vi "Exporting_last_uploaded_settings_Core.vi"() -> ()   [LabVIEW 2011]
uses:
  common/typedefs/Waveforms_Cluster_Core.ctl
  common/typedefs/Unit_Names_Core.ctl
  common/typedefs/Data_Sources_Core.ctl
  common/typedefs/Types_of_Signals_Core.ctl
  common/typedefs/Types_of_Analyses_Core.ctl
  common/typedefs/Analysis_Parameters_Cluster_Core.ctl
  <vilib>/Analysis/3filter.llb/Filter Passband Type.ctl
  common/typedefs/Integration_Types_Core.ctl
  common/typedefs/Pan_Cluster_Core.ctl
  common/typedefs/Condition_Vector_Cluster_Core.ctl
  common/typedefs/cRIO_System_Settings_Cluster_Core.ctl
  common/typedefs/DSA_Channels_Configuration_Core.ctl
  <vilib>/addons/database/Connection.llb/DB Tools Open Connec (String).vi
  <vilib>/addons/database/Connection.llb/Conn Execute.vi
  <vilib>/addons/database/Recordset.llb/Rec Fetch Recordset Data (R).vi
  <vilib>/addons/database/Recordset.llb/Rec Destroy - Connection.vi
  <vilib>/addons/database/_DB Variant To Data/Database Variant To Data.xnode
  <vilib>/addons/database/NI_Database_API.lvlib
  <vilib>/Analysis/NI_AALBase.lvlib
panel:
  out "SettingsDescription (Always) 4":string
  out "Timestamp (Always) 4":dbl
  out "idtsettings (Always) 4":u32
  out "error out 10":errorcluster
  out "error out 9":errorcluster
  in  "cRIO system settings cluster 2":T1={"CONFIG Folder - Relative Path "=path "", "FIFO Depth (# of elements)"=0, "Avoid ALARM/ TRIP in transient regimes?"=FALSE, "Sample Rate [Hz]"=0.0, "Processing interval [s]"=0.0, "Total number of channels to read from FPGA  (auto-calculated)"=0, "# of data to read-DMA (auto-calculated)"=0, "SysLog Interval (s)"=0, "Running Log Folder - Relative Path "=path "Logs/Running_Log", "Reset Log File - Relative Path "=path "Logs/ResetLogs/cRIO_reset.txt", "Error Log File - Relative Path "=path "Logs/ErrLogs/Errlogs.txt", "Ring Buffer Size (# Log File Elements)"=86400, "CPU Usage Exceed Limit ()"=98.0, "CPU Usage Exceed Limit Delay (# of iterrations)"=60, "Free Memory Min Avail.  (%)"=15.0, "Base CoDiS Folder"=path "c:/CoDiS", "Archive Log Folder - Relative Path "=path "Logs/Archive_Log", "Avail. Drive Space Limit to do Archive (%)"=20.0, "Mediator IP address"="10.50.10.1", "Mediator Communication TCP/IP Port"=2055, "Used channels (from FPGA) per units -Auto calculated"=[], "# DMA FIFO Fulls File - Relative Path "=path "Logs/ResetLogs/cRIO_reset.txt", "Log Status Parameters in cRIO Ring Buffer"=FALSE, "Channels Input Configuration (has to be defined for all available AI)"=[], "Index to check OL and SC (from FPGA) per units and channels -Auto calculated)"=[], "System not OK? (Auto-calculated)"=FALSE, "System not OK Relay Number (-1 = none, 0,..., MAX)"=-1, "Use normal (T) or inverse (F) relay logic for given relay (size of array equals to number of relays)?"=[], "U32 Relay Output (Auto-calculated)"=0, "cRIO Source"=enum."Not Used", "Check DMA FIFO Full?"=FALSE, "Modbus Settings"={"Modbus Communication Port"=502, "Run as Modbus Server/Slave? (FALSE=Modbus Client/Master)"=FALSE, "Modbus Slave Remote IP Address (if Run as Modbus Server/Slave?=FALSE)"=""}, "Time Synchronization Settings"={"Enable Time Synchronization"=FALSE, "Time Server IP Address (if Enable Time Synchronization=TRUE)"=""}} {"Channels Input Configuration (has to be defined for all available AI)" items=["AC Coupled", "DC Coupled", "IEPE AC Coupled", "Not DSA Channel"]}
  in  "cRIO system settings cluster":T1={"CONFIG Folder - Relative Path "=path "", "FIFO Depth (# of elements)"=0, "Avoid ALARM/ TRIP in transient regimes?"=FALSE, "Sample Rate [Hz]"=0.0, "Processing interval [s]"=0.0, "Total number of channels to read from FPGA  (auto-calculated)"=0, "# of data to read-DMA (auto-calculated)"=0, "SysLog Interval (s)"=0, "Running Log Folder - Relative Path "=path "Logs/Running_Log", "Reset Log File - Relative Path "=path "Logs/ResetLogs/cRIO_reset.txt", "Error Log File - Relative Path "=path "Logs/ErrLogs/Errlogs.txt", "Ring Buffer Size (# Log File Elements)"=86400, "CPU Usage Exceed Limit ()"=98.0, "CPU Usage Exceed Limit Delay (# of iterrations)"=60, "Free Memory Min Avail.  (%)"=15.0, "Base CoDiS Folder"=path "c:/CoDiS", "Archive Log Folder - Relative Path "=path "Logs/Archive_Log", "Avail. Drive Space Limit to do Archive (%)"=20.0, "Mediator IP address"="10.50.10.1", "Mediator Communication TCP/IP Port"=2055, "Used channels (from FPGA) per units -Auto calculated"=[], "# DMA FIFO Fulls File - Relative Path "=path "Logs/ResetLogs/cRIO_reset.txt", "Log Status Parameters in cRIO Ring Buffer"=FALSE, "Channels Input Configuration (has to be defined for all available AI)"=[], "Index to check OL and SC (from FPGA) per units and channels -Auto calculated)"=[], "System not OK? (Auto-calculated)"=FALSE, "System not OK Relay Number (-1 = none, 0,..., MAX)"=-1, "Use normal (T) or inverse (F) relay logic for given relay (size of array equals to number of relays)?"=[], "U32 Relay Output (Auto-calculated)"=0, "cRIO Source"=enum."Not Used", "Check DMA FIFO Full?"=FALSE, "Modbus Settings"={"Modbus Communication Port"=502, "Run as Modbus Server/Slave? (FALSE=Modbus Client/Master)"=FALSE, "Modbus Slave Remote IP Address (if Run as Modbus Server/Slave?=FALSE)"=""}, "Time Synchronization Settings"={"Enable Time Synchronization"=FALSE, "Time Server IP Address (if Enable Time Synchronization=TRUE)"=""}} {"Channels Input Configuration (has to be defined for all available AI)" items=["AC Coupled", "DC Coupled", "IEPE AC Coupled", "Not DSA Channel"]}
  in  "Pan Cluster":T4={"Configuration File loaded successfully?"=FALSE, "Is this new configuration?"=FALSE, "Condition Vector Cluster"={"Unit Name"=enum."Unit 2", "Source Name"=[], "Use CoDiS server Timestamp (on FALSE uses Processing Unit Timestamp)?"=FALSE, "Timestamp (DBL)"=0.0, "Mode of Operation - Normal (Settings)"=[], "Mode of Operation - Normal"="", "Mode of Operation - Diagnostic (Settings)"=[], "Mode of Operation - Diagnostic Recognized Index"=0, "Condition Vector Label"=[], "Condition Vector Name"=[], "Is this Main Trigger Signal?"=[], "Perform PRE-ALARM, ALARM, etc. Analysis on CoDiS server (mediator main calc. loop)?"=[], "Trigger Indexes"=[], "Condition Vector Values Complex (CDB)"=[], "Condition Vector Values"=[], "Save to dBase"=[], "Check if Condition Vector Element is out of Range"=[], "Condition Vector Low Limit Value"=[], "Condition Vector High Limit Value"=[], "Condition Vector Element out of Range"=[], "Check for PRE-ALARM"=[], "PRE-ALARM Value"=[], "Number of Loops in PRE-ALARM"=[], "PRE-ALARM Delay in # of Loops"=[], "Is Value Increasing for PRE-ALARM?"=[], "In PRE-ALARM?"=[], "In Delayed PRE-ALARM?"=[], "In Delayed PRE-ALARM REM?"=[], "Save PRE-ALARM?"=FALSE, "Check for ALARM"=[], "ALARM Value"=[], "Number of Loops in ALARM"=[], "ALARM Delay in # of Loops"=[], "Is Value Increasing for ALARM?"=[], "In ALARM?"=[], "In Delayed ALARM?"=[], "In Delayed ALARM REM?"=[], "Save ALARM?"=FALSE, "ALARM Relay Number (-1 = none, 0, ..., MAX)"=[], "Check for PRE-TRIP"=[], "PRE-TRIP Value"=[], "Number of Loops in PRE-TRIP"=[], "PRE-TRIP Delay in # of Loops"=[], "Is Value Increasing for PRE-TRIP?"=[], "In PRE-TRIP?"=[], "In Delayed PRE-TRIP?"=[], "In Delayed PRE-TRIP REM?"=[], "Save PRE-TRIP?"=FALSE, "Check for TRIP"=[], "TRIP Value"=[], "Number of Loops in TRIP"=[], "TRIP Delay in # of Loops"=[], "Is Value Increasing for TRIP?"=[], "In TRIP?"=[], "In Delayed TRIP?"=[], "In Delayed TRIP REM?"=[], "Save TRIP?"=FALSE, "TRIP Relay Number(-1 = none, 0,..., MAX)"=[], "Check for Diagnostic ALARM"=[], "ZERO Machine Signature Value"=[], "Number of Loops in Diagnostic ALARM"=[], "Diagnostic ALARM Delay in # of Loops"=[], "Is Value Increasing for Diagnostic ALARM?"=[], "In Diagnostic ALARM?"=[], "In Delayed Diagnostic ALARM?"=[], "In Delayed Diagnostic ALARM REM?"=[], "Save Diagnostic ALARM?"=FALSE, "Current Diagnostic Alarm Level"=[], "Delta for Diagnostic ALARM"=[], "Trigger RS for this channel?"=[], "Delta for RS Trigger"=[], "Modbus Parameters"={"Type"=[], "Modbus register"=[], "Which element type"=[], "Starting address"=[], "How many registers"=[], "Multiplication factor"=[]}, "Filter State"=[], "Apply Formula?"=[], "Formula Settings (If Apply Formula?=TRUE)"=[]}, "Orbit(s) - XY"=[], "Air Gap Data"=[], "Magnetic Field Data"=[], "Absolute Minimum Air Gap per Plane"=[]} {"Absolute Minimum Air Gap per Plane"."Absolute AG Minimum Pole Number" format="%.3f"; "Absolute Minimum Air Gap per Plane"."Absolute AG Minimum Value" format="%.3f"; "Magnetic Field Data"."Maximum by Pole Number" format="%.3f"; "Air Gap Data"."Minimum by Pole Number" format="%.3f"; "Orbit(s) - XY"."Orbit XY Graphs (Synthesized from Selected Harmonics and DC)"."?" format="%.3f"; "Orbit(s) - XY"."Orbit XY Graphs (Synthesized from Selected Harmonics and DC)"."?" format="%.3f"; "Orbit(s) - XY"."Orbit XY Graphs (Glided and Averaged on One Revolution)"."?" format="%.3f"; "Orbit(s) - XY"."Orbit XY Graphs (Glided and Averaged on One Revolution)"."?" format="%.3f"; "Orbit(s) - XY"."Orbit XY Graphs (Unaveraged)"."?" format="%.3f"; "Orbit(s) - XY"."Orbit XY Graphs (Unaveraged)"."?" format="%.3f"}
  out "error out 6":errorcluster
  out "error out 5":errorcluster
  out "idtsettings (Always) 3":u32
  out "Timestamp (Always) 3":dbl
  out "SettingsDescription (Always) 3":string
  out "error out 4":errorcluster
  out "error out 3":errorcluster
  out "idtsettings (Always) 2":u32
  out "Timestamp (Always) 2":dbl
  out "SettingsDescription (Always) 2":string
  out "error out 2":errorcluster
  out "error out":errorcluster
  in  "Empty Waveform Cluster":T7={"Configuration File loaded successfully? "=FALSE, "Is this new configuration?"=FALSE, "Unit Name"=enum."Unit 1", "Waveform Source"=[], "Use CoDiS server Timestamp (on FALSE uses Processing Unit Timestamp)?"=FALSE, "Sampling Rate [Hz]"=[], "Timestamp (DBL)"=0.0, "Mode of Operation - Normal"="", "Mode of Operation - Diagnostic"="", "Waveform Physical Channel"=[], "Waveform Label"=[], "Waveform Name"=[], "Signal Type"=[], "Is this Main Trigger Signal?"=[], "Slope"=[], "Intercept"=[], "Waveform Values"=[], "Analyse?"=[], "Save to database?"=[], "Analyses to Perform"=[], "Perform this analysis on a CoDiS server?"=[], "General Parameters"={"Number of Poles"=0, "Grid Frequency"=0.0}, "Analysis Parameters"=[], "Save now to dBase?"=FALSE, "Waveform Length for Saving [s]"=0, "Pretrigger Length when Saving Waveform [s]"=0, "Next Timestamp to autosave at (DBL)"=0.0, "Description of Waveforms Events"="", "Event Type"="", "Save next RS event entirely? (on FALSE uses How many basic (acquisition) blocks of data (loops) to save?"=FALSE, "Regime Name for which to save next RS event entirely"="", "Integration type"=[], "Channel not OK?"=[], "Channel Not OK?  Relay Number (-1 = none, 0, ..., MAX)"=[], "Array of FPGA Filter Parameters"=[], "Pre-Alarm Delay in Number of Loops "=0, "Pre-Trip Delay in Number of Loops "=0} {"Analysis Parameters"."SP2Pmax"."Filter Parameters"."low cutoff freq: fl" format="%0.4f"; "Analysis Parameters"."SP2Pmax"."Filter Parameters"."high cutoff freq: fh" format="%0.2f"; "Analysis Parameters"."LoadAngleDelta"."Multiplication Factor" format="%.1f"; "Analysis Parameters"."LoadAngleDelta"."What harmonic? (for example 24th (48 pole machine))" format="%.1f"; "Analysis Parameters"."Peak2Peak"."Filter Parameters"."low cutoff freq: fl" format="%0.4f"; "Analysis Parameters"."Peak2Peak"."Filter Parameters"."high cutoff freq: fh" format="%0.2f"; "Analysis Parameters"."RMS"."Filter Parameters"."order" format="%0.4f"; "Analysis Parameters"."RMS"."Filter Parameters"."low cutoff freq: fl" format="%0.2f"; "Analysis Parameters"."RMS"."Filter Parameters"."high cutoff freq: fh" format="%0.2f"; "Analysis Parameters"."EqPeak"."Filter Parameters"."low cutoff freq: fl" format="%0.4f"; "Analysis Parameters"."EqPeak"."Filter Parameters"."high cutoff freq: fh" format="%0.2f"; "Analysis Parameters"."Peak"."Filter Parameters"."low cutoff freq: fl" format="%0.4f"; "Analysis Parameters"."Peak"."Filter Parameters"."high cutoff freq: fh" format="%0.2f"; "Analysis Parameters"."snPh"."What harmonic?" format="%.1f"; "Analysis Parameters"."snA"."Multiplication Factor" format="%.1f"; "Analysis Parameters"."snA"."What harmonic?" format="%.1f"; "Analysis Parameters"."Smax"."Filter Parameters"."low cutoff freq: fl" format="%0.4f"; "Analysis Parameters"."Smax"."Filter Parameters"."high cutoff freq: fh" format="%0.2f"; "Analysis Parameters"."RPM"."Signal Threshold" format="%.1f"}
  out "idtsettings (Always)":u32
  out "Timestamp (Always)":dbl
  out "SettingsDescription (Always)":string
  out "Waveform Cluster (Depending on Selection)":T7={"Configuration File loaded successfully? "=FALSE, "Is this new configuration?"=FALSE, "Unit Name"=enum."Unit 1", "Waveform Source"=[], "Use CoDiS server Timestamp (on FALSE uses Processing Unit Timestamp)?"=FALSE, "Sampling Rate [Hz]"=[], "Timestamp (DBL)"=0.0, "Mode of Operation - Normal"="", "Mode of Operation - Diagnostic"="", "Waveform Physical Channel"=[], "Waveform Label"=[], "Waveform Name"=[], "Signal Type"=[], "Is this Main Trigger Signal?"=[], "Slope"=[], "Intercept"=[], "Waveform Values"=[], "Analyse?"=[], "Save to database?"=[], "Analyses to Perform"=[], "Perform this analysis on a CoDiS server?"=[], "General Parameters"={"Number of Poles"=0, "Grid Frequency"=0.0}, "Analysis Parameters"=[], "Save now to dBase?"=FALSE, "Waveform Length for Saving [s]"=0, "Pretrigger Length when Saving Waveform [s]"=0, "Next Timestamp to autosave at (DBL)"=0.0, "Description of Waveforms Events"="", "Event Type"="", "Save next RS event entirely? (on FALSE uses How many basic (acquisition) blocks of data (loops) to save?"=FALSE, "Regime Name for which to save next RS event entirely"="", "Integration type"=[], "Channel not OK?"=[], "Channel Not OK?  Relay Number (-1 = none, 0, ..., MAX)"=[], "Array of FPGA Filter Parameters"=[], "Pre-Alarm Delay in Number of Loops "=0, "Pre-Trip Delay in Number of Loops "=0} {"Analysis Parameters"."SP2Pmax"."Filter Parameters"."low cutoff freq: fl" format="%0.4f"; "Analysis Parameters"."SP2Pmax"."Filter Parameters"."high cutoff freq: fh" format="%0.2f"; "Analysis Parameters"."LoadAngleDelta"."Multiplication Factor" format="%.1f"; "Analysis Parameters"."LoadAngleDelta"."What harmonic? (for example 24th (48 pole machine))" format="%.1f"; "Analysis Parameters"."Peak2Peak"."Filter Parameters"."low cutoff freq: fl" format="%0.4f"; "Analysis Parameters"."Peak2Peak"."Filter Parameters"."high cutoff freq: fh" format="%0.2f"; "Analysis Parameters"."RMS"."Filter Parameters"."order" format="%0.4f"; "Analysis Parameters"."RMS"."Filter Parameters"."low cutoff freq: fl" format="%0.2f"; "Analysis Parameters"."RMS"."Filter Parameters"."high cutoff freq: fh" format="%0.2f"; "Analysis Parameters"."EqPeak"."Filter Parameters"."low cutoff freq: fl" format="%0.4f"; "Analysis Parameters"."EqPeak"."Filter Parameters"."high cutoff freq: fh" format="%0.2f"; "Analysis Parameters"."Peak"."Filter Parameters"."low cutoff freq: fl" format="%0.4f"; "Analysis Parameters"."Peak"."Filter Parameters"."high cutoff freq: fh" format="%0.2f"; "Analysis Parameters"."snPh"."What harmonic?" format="%.1f"; "Analysis Parameters"."snA"."Multiplication Factor" format="%.1f"; "Analysis Parameters"."snA"."What harmonic?" format="%.1f"; "Analysis Parameters"."Smax"."Filter Parameters"."low cutoff freq: fl" format="%0.4f"; "Analysis Parameters"."Smax"."Filter Parameters"."high cutoff freq: fh" format="%0.2f"; "Analysis Parameters"."RPM"."Signal Threshold" format="%.1f"}
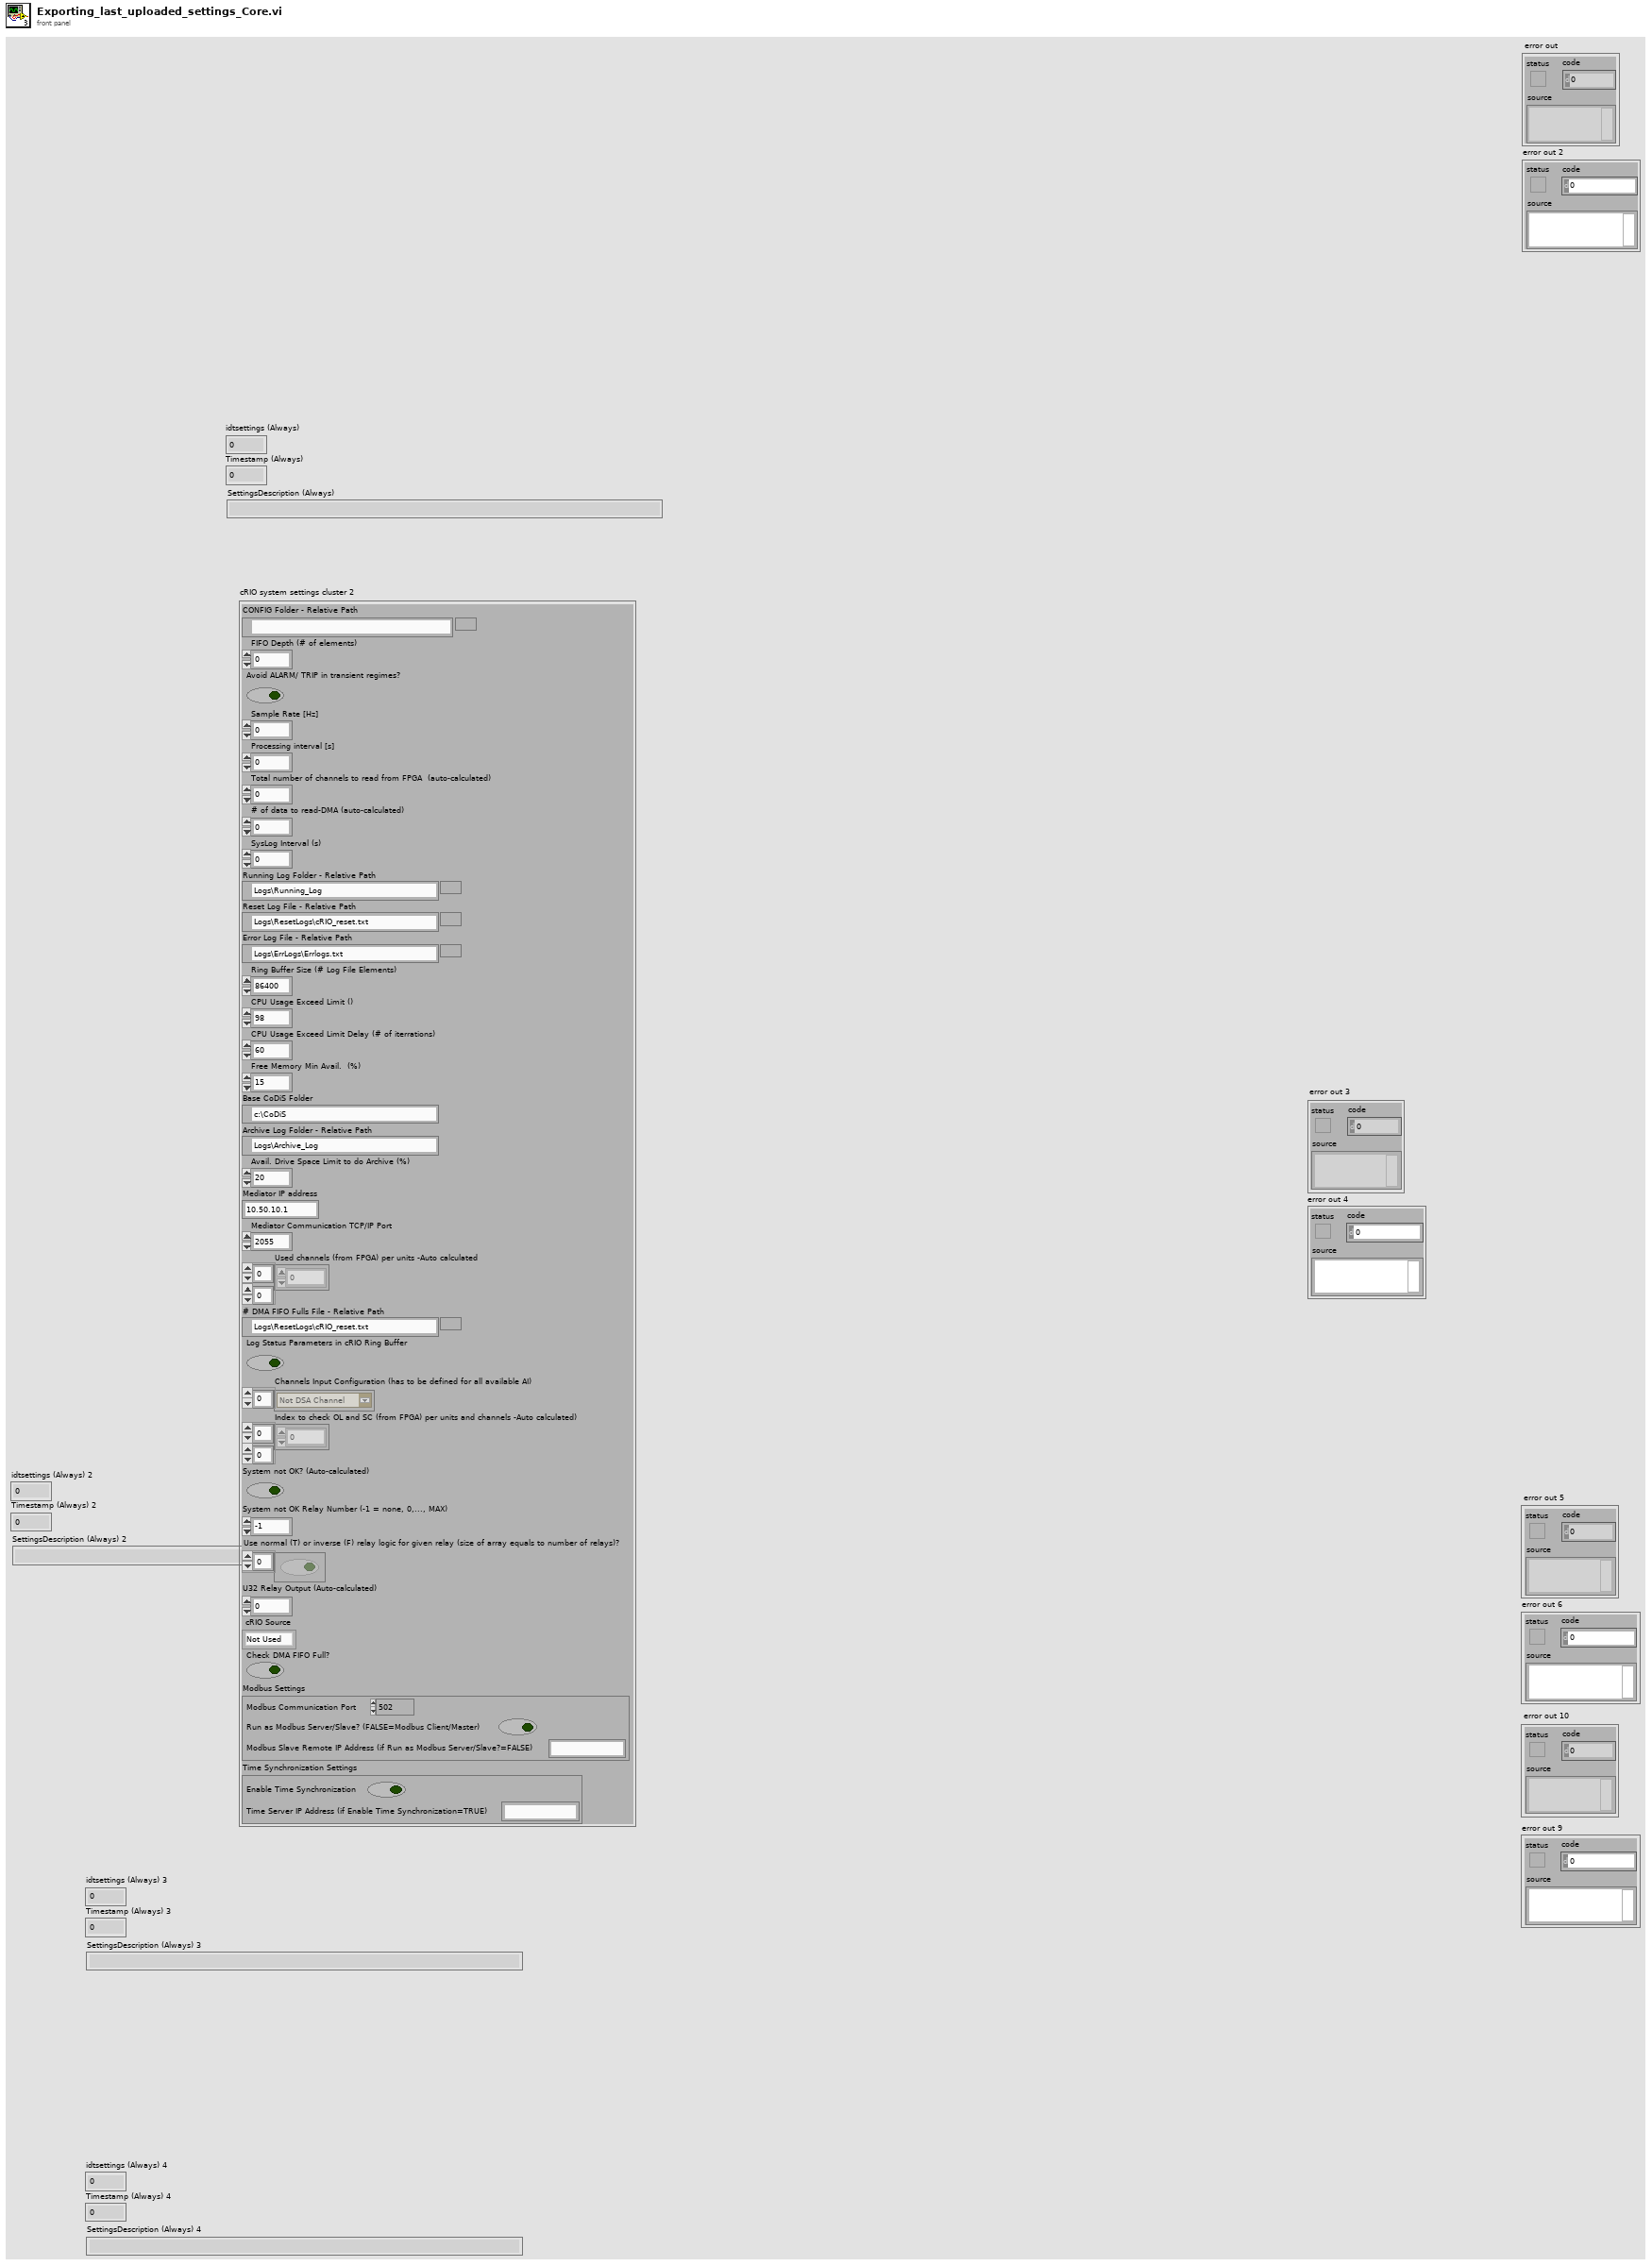
[diagram p1: front panel]
types:
  T1 = typedef "cRIO_System_Settings_Cluster_Core.ctl" = cluster{"CONFIG Folder - Relative Path ":path, "FIFO Depth (# of elements)":u32, "Avoid ALARM/ TRIP in transient regimes?":bool, "Sample Rate [Hz]":sgl, "Processing interval [s]":sgl, "Total number of channels to read from FPGA  (auto-calculated)":u32, "# of data to read-DMA (auto-calculated)":u32, "SysLog Interval (s)":u32, "Running Log Folder - Relative Path ":path, "Reset Log File - Relative Path ":path, "Error Log File - Relative Path ":path, "Ring Buffer Size (# Log File Elements)":u32, "CPU Usage Exceed Limit ()":sgl, "CPU Usage Exceed Limit Delay (# of iterrations)":u32, "Free Memory Min Avail.  (%)":sgl, "Base CoDiS Folder":path, "Archive Log Folder - Relative Path ":path, "Avail. Drive Space Limit to do Archive (%)":sgl, "Mediator IP address":string, "Mediator Communication TCP/IP Port":u16, "Used channels (from FPGA) per units -Auto calculated":i32[][], "# DMA FIFO Fulls File - Relative Path ":path, "Log Status Parameters in cRIO Ring Buffer":bool, "Channels Input Configuration (has to be defined for all available AI)":T2[], "Index to check OL and SC (from FPGA) per units and channels -Auto calculated)":i32[][], "System not OK? (Auto-calculated)":bool, "System not OK Relay Number (-1 = none, 0,..., MAX)":i16, "Use normal (T) or inverse (F) relay logic for given relay (size of array equals to number of relays)?":bool[], "U32 Relay Output (Auto-calculated)":u32, "cRIO Source":T3, "Check DMA FIFO Full?":bool, "Modbus Settings":cluster{"Modbus Communication Port":u16, "Run as Modbus Server/Slave? (FALSE=Modbus Client/Master)":bool, "Modbus Slave Remote IP Address (if Run as Modbus Server/Slave?=FALSE)":string}, "Time Synchronization Settings":cluster{"Enable Time Synchronization":bool, "Time Server IP Address (if Enable Time Synchronization=TRUE)":string}}
  T2 = typedef "DSA_Channels_Configuration_Core.ctl" = u16
  T3 = typedef "Data_Sources_Core.ctl" = enum16{"Not Used", "Source 0", "Source 1", "Source 2", "Source 3", "Source 4", "Source 5", "Source 6", "Source 7", "Source 8", "Source 9", "Source 10", "Source 11", "Source 12", "Source 13", "Source 14", "Source 15", "Source 16", "Source 17", "Source 18", "Source 19", "Source 20"}
  T4 = typedef "Pan_Cluster_Core.ctl" = cluster{"Configuration File loaded successfully?":bool, "Is this new configuration?":bool, "Condition Vector Cluster":T5, "Orbit(s) - XY":cluster{"Bearing Plane Label (for example RV000&RV001 or RV001&RV000; 1st label is X, second is Y)":string, "Bearing Plane Name (for client purposes)":string, "Orbit XY Graphs (Unaveraged)":cluster{sgl[], sgl[]}[], "Glided and Averaged on One Revolution Parameters Cluster":cluster{"Calculate from time-averaged signal on one revolution?":bool, "Analyze data from 1st trigger to last (if possible)? (FALSE=analyze everything)":bool, "Gliding Parameters":cluster{"Glide signal?":bool, "Number of points for gliding":u16}}, "Orbit XY Graphs (Glided and Averaged on One Revolution)":cluster{sgl[], sgl[]}[], "Orbit XY Graphs (Synthesized from Selected Harmonics and DC)":cluster{sgl[], sgl[]}[], "Rotate Coordinate System?":bool, "Angle for rot. (if Rotate Coordinate System?=TRUE; angle is >0 for CCW, <0 for CW - view from generator (above for vert. mach.) side)":sgl}[], "Air Gap Data":cluster{"Air Gap Label":string, "Minimum by Pole Number":sgl[]}[], "Magnetic Field Data":cluster{"Magnetic Field Label":string, "Maximum by Pole Number":sgl[]}[], "Absolute Minimum Air Gap per Plane":cluster{"Air Gap Plane Name":string, "Air Gap Sensor Labels per Plane":string[], "Air Gap Sensor Name per Plane":string[], "Absolute AG Minimum Value":sgl, "Absolute AG Minimum Pole Number":sgl, "Absolute AG Minimum Sensor Label":string, "Absolute AG Minimum Sensor Name":string}[]}
  T5 = typedef "Condition_Vector_Cluster_Core.ctl" = cluster{"Unit Name":T6, "Source Name":T3[], "Use CoDiS server Timestamp (on FALSE uses Processing Unit Timestamp)?":bool, "Timestamp (DBL)":dbl, "Mode of Operation - Normal (Settings)":cluster{"Regime Name":string, "Regime Logical Definition Statement":string}[], "Mode of Operation - Normal":string, "Mode of Operation - Diagnostic (Settings)":cluster{"Regime Name":string, "Regime Logical Definition Statement":string}[], "Mode of Operation - Diagnostic Recognized Index":i16, "Condition Vector Label":string[], "Condition Vector Name":string[], "Is this Main Trigger Signal?":bool[], "Perform PRE-ALARM, ALARM, etc. Analysis on CoDiS server (mediator main calc. loop)?":bool[], "Trigger Indexes":u32[], "Condition Vector Values Complex (CDB)":cdb[], "Condition Vector Values":sgl[], "Save to dBase":bool[], "Check if Condition Vector Element is out of Range":bool[], "Condition Vector Low Limit Value":sgl[], "Condition Vector High Limit Value":sgl[], "Condition Vector Element out of Range":bool[], "Check for PRE-ALARM":bool[][], "PRE-ALARM Value":sgl[][], "Number of Loops in PRE-ALARM":u32[], "PRE-ALARM Delay in # of Loops":u16[][], "Is Value Increasing for PRE-ALARM?":bool[], "In PRE-ALARM?":bool[], "In Delayed PRE-ALARM?":bool[], "In Delayed PRE-ALARM REM?":bool[], "Save PRE-ALARM?":bool, "Check for ALARM":bool[][], "ALARM Value":sgl[][], "Number of Loops in ALARM":u32[], "ALARM Delay in # of Loops":u16[][], "Is Value Increasing for ALARM?":bool[], "In ALARM?":bool[], "In Delayed ALARM?":bool[], "In Delayed ALARM REM?":bool[], "Save ALARM?":bool, "ALARM Relay Number (-1 = none, 0, ..., MAX)":i16[], "Check for PRE-TRIP":bool[][], "PRE-TRIP Value":sgl[][], "Number of Loops in PRE-TRIP":u32[], "PRE-TRIP Delay in # of Loops":u16[][], "Is Value Increasing for PRE-TRIP?":bool[], "In PRE-TRIP?":bool[], "In Delayed PRE-TRIP?":bool[], "In Delayed PRE-TRIP REM?":bool[], "Save PRE-TRIP?":bool, "Check for TRIP":bool[][], "TRIP Value":sgl[][], "Number of Loops in TRIP":u32[], "TRIP Delay in # of Loops":u16[][], "Is Value Increasing for TRIP?":bool[], "In TRIP?":bool[], "In Delayed TRIP?":bool[], "In Delayed TRIP REM?":bool[], "Save TRIP?":bool, "TRIP Relay Number(-1 = none, 0,..., MAX)":i16[], "Check for Diagnostic ALARM":bool[][], "ZERO Machine Signature Value":dbl[][], "Number of Loops in Diagnostic ALARM":u32[], "Diagnostic ALARM Delay in # of Loops":u16[][], "Is Value Increasing for Diagnostic ALARM?":bool[], "In Diagnostic ALARM?":bool[], "In Delayed Diagnostic ALARM?":bool[], "In Delayed Diagnostic ALARM REM?":bool[], "Save Diagnostic ALARM?":bool, "Current Diagnostic Alarm Level":sgl[][], "Delta for Diagnostic ALARM":sgl[][], "Trigger RS for this channel?":bool[][], "Delta for RS Trigger":sgl[][], "Modbus Parameters":cluster{"Type":enum16{"Read", "Write", "None"}[][], "Modbus register":enum16{"Coils", "Discrete Inputs", "Input Registers", "Holding Registers"}[][], "Which element type":enum16{"Value", "Alarm", "Trip"}[][], "Starting address":u16[][], "How many registers":enum16{"Single register", "HI-LO", "LO-HI"}[][], "Multiplication factor":dbl[][]}, "Filter State":cluster{"Filter State (channels by rows: 0. ch0, 1. ch1, etc))":dbl[][]}[], "Apply Formula?":bool[][], "Formula Settings (If Apply Formula?=TRUE)":cluster{"Variables by Condition vector label (Example (array):  0. PROC000.DC; 1.PROC001.DC000)":string[], "Formula (example: (PROC000.DC+PROC001.DC000)/2  )":string}[][]}
  T6 = typedef "Unit_Names_Core.ctl" = enum16{"Not used", "Unit 1", "Unit 2", "Unit 3", "Unit 4", "Unit 5", "Unit 6", "Unit 7", "Unit 8", "Unit 9"}
  T7 = typedef "Waveforms_Cluster_Core.ctl" = cluster{"Configuration File loaded successfully? ":bool, "Is this new configuration?":bool, "Unit Name":T6, "Waveform Source":T3[], "Use CoDiS server Timestamp (on FALSE uses Processing Unit Timestamp)?":bool, "Sampling Rate [Hz]":u32[], "Timestamp (DBL)":dbl, "Mode of Operation - Normal":string, "Mode of Operation - Diagnostic":string, "Waveform Physical Channel":u16[], "Waveform Label":string[], "Waveform Name":string[], "Signal Type":cluster{"Signal Type":T8, "# of signal of particular type":u8}[], "Is this Main Trigger Signal?":bool[], "Slope":dbl[], "Intercept":dbl[], "Waveform Values":sgl[][], "Analyse?":bool[], "Save to database?":bool[], "Analyses to Perform":T9[][], "Perform this analysis on a CoDiS server?":bool[][], "General Parameters":cluster{"Number of Poles":u8, "Grid Frequency":sgl}, "Analysis Parameters":T10[][], "Save now to dBase?":bool, "Waveform Length for Saving [s]":u16, "Pretrigger Length when Saving Waveform [s]":u16, "Next Timestamp to autosave at (DBL)":dbl, "Description of Waveforms Events":string, "Event Type":string, "Save next RS event entirely? (on FALSE uses How many basic (acquisition) blocks of data (loops) to save?":bool, "Regime Name for which to save next RS event entirely":string, "Integration type":T12[], "Channel not OK?":bool[], "Channel Not OK?  Relay Number (-1 = none, 0, ..., MAX)":i16[], "Array of FPGA Filter Parameters":cluster{"Filter signal?":bool, "filter type":T11, "high cutoff freq: fh":dbl, "low cutoff freq: fl":dbl, "order":i32}[][], "Pre-Alarm Delay in Number of Loops ":u16, "Pre-Trip Delay in Number of Loops ":u16}
  T8 = typedef "Types_of_Signals_Core.ctl" = enum16{"Not Used", "Trigger (TRG???)", "Relative Vibrations (RV???)", "Absolute Vibrations (AV???)", "Air Gap (AG???)", "Magnetic Field (MX???)", "Voltage (VOL???)", "Current (CURR???)", "Process (PROC???)", "Cavitation (CAV???)", "Non Standard (NONST???)", "Axial Displacement (AXD???)", "Absolute Vibrations Stator Core (AVSC???)"}
  T9 = typedef "Types_of_Analyses_Core.ctl" = enum16{"Exit Analysis Loop", "Do Nothing", "RPM", "Smax", "SP2Pmax", "snA", "snPh", "Rest", "Peak", "EqPeak", "Peak2Peak", "RMS", "DC", "DC from Extrema", "Min Value", "Max Value", "Min Value by Pole", "Max Value by Pole", "Max Diff by Pole", "Max Diff Pole Number", "Min from Extrema", "Max from Extrema", "Active Power from DFT", "Active Power by Integration", "Reactive Power from DFT", "Reactive Power by Integration", "Apparent Power", "Ampl@Freq", "Phase Difference", "Load Angle Delta", "THD", "Signal Frequency", "Eta", "Non standard (CoDiS server - manual) 0", "Non standard (CoDiS server - manual) 1", "Non standard (CoDiS server - manual) 2", "Non standard (CoDiS server - manual) 3", "Non standard (CoDiS server - manual) 4", "Non standard (CoDiS server - manual) 5", "Non standard (CoDiS server - manual) 6", "Non standard (CoDiS server - manual) 7", "Non standard (CoDiS server - manual) 8", "Non standard (CoDiS server - manual) 9", "Non standard (CoDiS server - manual) 10", "Non standard (CoDiS server - manual) 11", "Non standard (CoDiS server - manual) 12", "Non standard (CoDiS server - manual) 13", "Non standard (CoDiS server - manual) 14", "Non standard (CoDiS server - manual) 15", "Non standard (CoDiS server - manual) 16", "Non standard (CoDiS server - manual) 17", "Non standard (CoDiS server - manual) 18", "Non standard (CoDiS server - manual) 19", "CosFi", "Total THD", "Crest Factor"}
  T10 = typedef "Analysis_Parameters_Cluster_Core.ctl" = cluster{"DC":cluster{"Analyze data from 1st trigger to last (if possible)? (FALSE=analyze everything)":bool}, "DCExtrema":cluster{"Calculate DC from all Pole Values":bool, "Poles to use in DC calculation (if Calculate DC from all Pole Values is FALSE)":u8[], "Condition Vector Label begin Part (MinPole or MaxPole)":string, "Addition to Condition Vector Label (example: 000)":string}, "RPM":cluster{"Signal Threshold":sgl, "Pulse Width (should be >= 2 depending on signal noise)":i32, "Trigger on rising edge? (FALSE=trigger on falling)":bool}, "Smax":cluster{"Combine with which Waveform Label? (for example: RV001)":string, "Calculate from time-averaged signal on one revolution?":bool, "Analyze data from 1st trigger to last (if possible)? (FALSE=analyze everything)":bool, "Filter Parameters":cluster{"Filter signal?":bool, "filter type":T11, "high cutoff freq: fh":dbl, "low cutoff freq: fl":dbl, "order":i32, "Process as ring-buffer signal?":bool}, "Gliding Parameters":cluster{"Glide signal?":bool, "Number of points for gliding":u16}, "Average all calculated values for Smax - if present (each revolution)? (FALSE=take absolute maximum)":bool, "Addition to Condition Vector Label (example: 000)":string}, "SP2Pmax":cluster{"Combine with which Waveform Label? (for example: RV001)":string, "Calculate from time-averaged signal on one revolution?":bool, "Analyze data from 1st trigger to last (if possible)? (FALSE=analyze everything)":bool, "Filter Parameters":cluster{"Filter signal?":bool, "filter type":T11, "high cutoff freq: fh":dbl, "low cutoff freq: fl":dbl, "order":i32, "Process as ring-buffer signal?":bool}, "Gliding Parameters":cluster{"Glide signal?":bool, "Number of points for gliding":u16}, "Average all calculated values for SP2Pmax - if present (each revolution)? (FALSE=take absolute maximum)":bool, "Addition to Condition Vector Label (example: 000)":string}, "snA":cluster{"What harmonic?":sgl, "Calculate Amplitude (TRUE) or RMS (FALSE)?":bool, "Multiplication Factor":sgl, "Calculate Amplitude for Air Gap type signals? (from MinPole Values)":bool}, "snPh":cluster{"What harmonic?":sgl}, "Peak":cluster{"Calculate from time-averaged signal (one-revolution)?":bool, "Analyze data from 1st trigger to last (if possible)? (FALSE=analyze everything)":bool, "Filter Parameters":cluster{"Filter signal?":bool, "filter type":T11, "high cutoff freq: fh":dbl, "low cutoff freq: fl":dbl, "order":i32, "Process as ring-buffer signal?":bool}, "Gliding Parameters":cluster{"Glide signal?":bool, "Number of points for gliding":u16}, "Average all calculated values for Peak - if present (each revolution)? (FALSE=take absolute maximum)":bool, "Addition to Condition Vector Label (example: 000)":string}, "Peak2Peak":cluster{"Calculate from time-averaged signal (one-revolution)?":bool, "Analyze data from 1st trigger to last (if possible)? (FALSE=analyze everything)":bool, "Gliding Parameters":cluster{"Glide signal?":bool, "Number of points for gliding":u16}, "Filter Parameters":cluster{"Filter signal?":bool, "filter type":T11, "high cutoff freq: fh":dbl, "low cutoff freq: fl":dbl, "order":i32, "Process as ring-buffer signal?":bool}, "Average all calculated values for Peak2Peak - if present (each revolution)? (FALSE=take absolute maximum)":bool, "Addition to Condition Vector Label (example: 000)":string}, "EqPeak":cluster{"Calculate from time-averaged signal (one-revolution)?":bool, "Analyze data from 1st trigger to last (if possible)? (FALSE=analyze everything)":bool, "Average all calculated values for EqPeak - if present (each revolution)? (FALSE=take absolute maximum)":bool, "Filter Parameters":cluster{"Filter signal?":bool, "filter type":T11, "high cutoff freq: fh":dbl, "low cutoff freq: fl":dbl, "order":i32, "Process as ring-buffer signal?":bool}, "Which Condition Vector Label addition to use for RMS (example: 001)":string, "Addition to Condition Vector Label (example: 000)":string}, "RMS":cluster{"Calculate from time-averaged signal (one-revolution)?":bool, "Analyze data from 1st trigger to last (if possible)? (FALSE=analyze everything)":bool, "Subtract DC before RMS calculation?":bool, "Filter Parameters":cluster{"Filter signal?":bool, "filter type":T11, "high cutoff freq: fh":dbl, "low cutoff freq: fl":dbl, "order":i32, "Process as ring-buffer signal?":bool}, "Gliding Parameters":cluster{"Glide signal?":bool, "Number of points for gliding":u16}, "Average all calculated values for RMS - if present (each revolution)? (FALSE=take absolute maximum)":bool, "Addition to Condition Vector Label (example: 000)":string}, "Rest":cluster{"Calculate from all calculated harmonics?":bool, "Condition Vector Label to use for substraction (if Calculate from all calculated harmonics?=FALSE)":string[], "Calculate by subtracting from EqPeak Value? (FALSE=calculate by subtracting from RMS Value)":bool, "Which Condition Vector Label addition to use for EqPeak (example: 001)":string, "Addition to Condition Vector Label (example: 000)":string}, "MinByPole":cluster{"First Pole Number after Trigger (indexes correspond to Normal regime settings)":u8[], "Are Pole Numbers in ascending order in time?  (indexes correspond to Normal regime settings)":bool[], "Average all calculated values for that Pole? (FALSE=take absolute minimum)":bool, "Coerce Upper Limit":sgl, "Compensate 1st harmonic in waveform?":bool}, "MinExtrema":cluster{"Calculate Min Extrema from all Pole Values":bool, "Poles to use in Min Extrema calculation (if Calculate Min Extrema from all Pole Values is FALSE)":u8[], "Condition Vector Label begin Part (MinPole or MaxPole)":string}, "MaxByPole":cluster{"First Pole Number after Trigger (indexes correspond to Normal regime settings)":u8[], "Are Pole Numbers in ascending order in time? (indexes correspond to Normal regime settings)":bool[], "Average all calculated values for that Pole? (FALSE=take absolute maximum)":bool, "Calculate with abs(Signal)?":bool, "Subtract DC before calculation?":bool, "Coerce Lower Limit":sgl}, "MaxExtrema":cluster{"Calculate Max Extrema from all Pole Values":bool, "Poles to use in Max Extrema calculation (if Calculate Max Extrema from all Pole Values is FALSE)":u8[], "Condition Vector Label begin Part (MinPole or MaxPole)":string}, "MaxDiffByPole":cluster{"First Pole Number after Trigger (indexes correspond to Normal regime settings)":u8[], "Are Pole Numbers in ascending order in time? (indexes correspond to Normal regime settings)":bool[], "Condition Vector Label begin Part (MinPole or MaxPole)":string}, "Min":cluster{"Analyze data from 1st trigger to last (if possible)? (FALSE=analyze everything)":bool, "Calculate from time-averaged signal on one revolution?":bool, "Gliding Parameters":cluster{"Glide signal?":bool, "Number of points for gliding":u16}, "Average all calculated values for Min - if present (each revolution)? (FALSE=take absolute maximum)":bool}, "Max":cluster{"Analyze data from 1st trigger to last (if possible)? (FALSE=analyze everything)":bool, "Calculate from time-averaged signal on one revolution?":bool, "Gliding Parameters":cluster{"Glide signal?":bool, "Number of points for gliding":u16}, "Average all calculated values for Max - if present (each revolution)? (FALSE=take absolute maximum)":bool}, "ActivePower":cluster{"Calculate from Phase Voltages and Currents?":bool, "Phase Voltage Condition Vector Label (R, S, T) (for example: VOL000.s24.00A, VOL001.s24.00A, VOL002.s24.00A)":string[], "Phase Current Condition Vector Label (R, S, T) (for example: CURR000.s24.00A, CURR001.s24.00A, CURR002.s24.00A)":string[]}, "ReactivePower":cluster{"Calculate from Phase Voltages and Currents?":bool, "Phase Voltage Condition Vector Label (R, S, T) (for example: VOL000.s24.00A, VOL001.s24.00A, VOL002.s24.00A)":string[], "Phase Current Condition Vector Label (R, S, T) (for example: CURR000.s24.00A, CURR001.s24.00A, CURR002.s24.00A)":string[]}, "LoadAngleDelta":cluster{"What harmonic? (for example 24th (48 pole machine))":sgl, "Delta0":sgl, "Which Voltage Waveform Label? (for example: VOL000)":string, "Combine (multiply) with which Air Gap Waveform Label? (for example: AG000)":string, "Multiplication Factor":sgl}, "ActivePowerByIntegration":cluster{"Phase Voltage Waveform Labels (R,S,T)":string[], "Phase Current Waveform Labels (R,S,T)":string[], "Analyze data from 1st trigger to last (if possible)? (FALSE=analyze everything)":bool}, "RectivePowerByIntegration":cluster{"Phase Voltage Waveform Vector Labels (R,S,T)":string[], "Phase Current Waveform Labels (R,S,T)":string[], "System Electric Frequency [Hz]":sgl, "Analyze data from 1st trigger to last (if possible)? (FALSE=analyze everything)":bool}, "Ampl@Freq":cluster{"Frequency [Hz]":sgl, "Calculate Amplitude? (FALSE=calculate RMS)":bool}, "PhaseDifference":cluster{"Combine with which Waveform Label?":string}, "CosFi":cluster{"Voltage Waveform Labels (R,S,T)":string[], "Current Waveform Labels (R,S,T)":string[]}, "Total THD":cluster{"THD Condition Vector Label (R, S, T) (for example: VOL000.THD, VOL001.THD, VOL002.THD)":string[]}, "Crest Factor":cluster{"Addition to Condition Vector Label (example: 000)":string, "Which Condition Vector Label addition to use for Peak (example: 001)":string, "Which Condition Vector Label addition to use for RMS (example: 001)":string}}
  T11 = typedef "NI_AALBase.lvlib/Filter Passband Type.ctl" = enum32{"Lowpass", "Highpass", "Bandpass", "Bandstop"}
  T12 = typedef "Integration_Types_Core.ctl" = enum16{"Do not integrate", "Integrate once", "Integrate twice"}
  T13 = typedef "NI_Database_API.lvlib/Conn ObjectReference.ctl" = refnum<k1>
  T14 = typedef "NI_Database_API.lvlib/Rec ObjectReference.ctl" = refnum<k1>
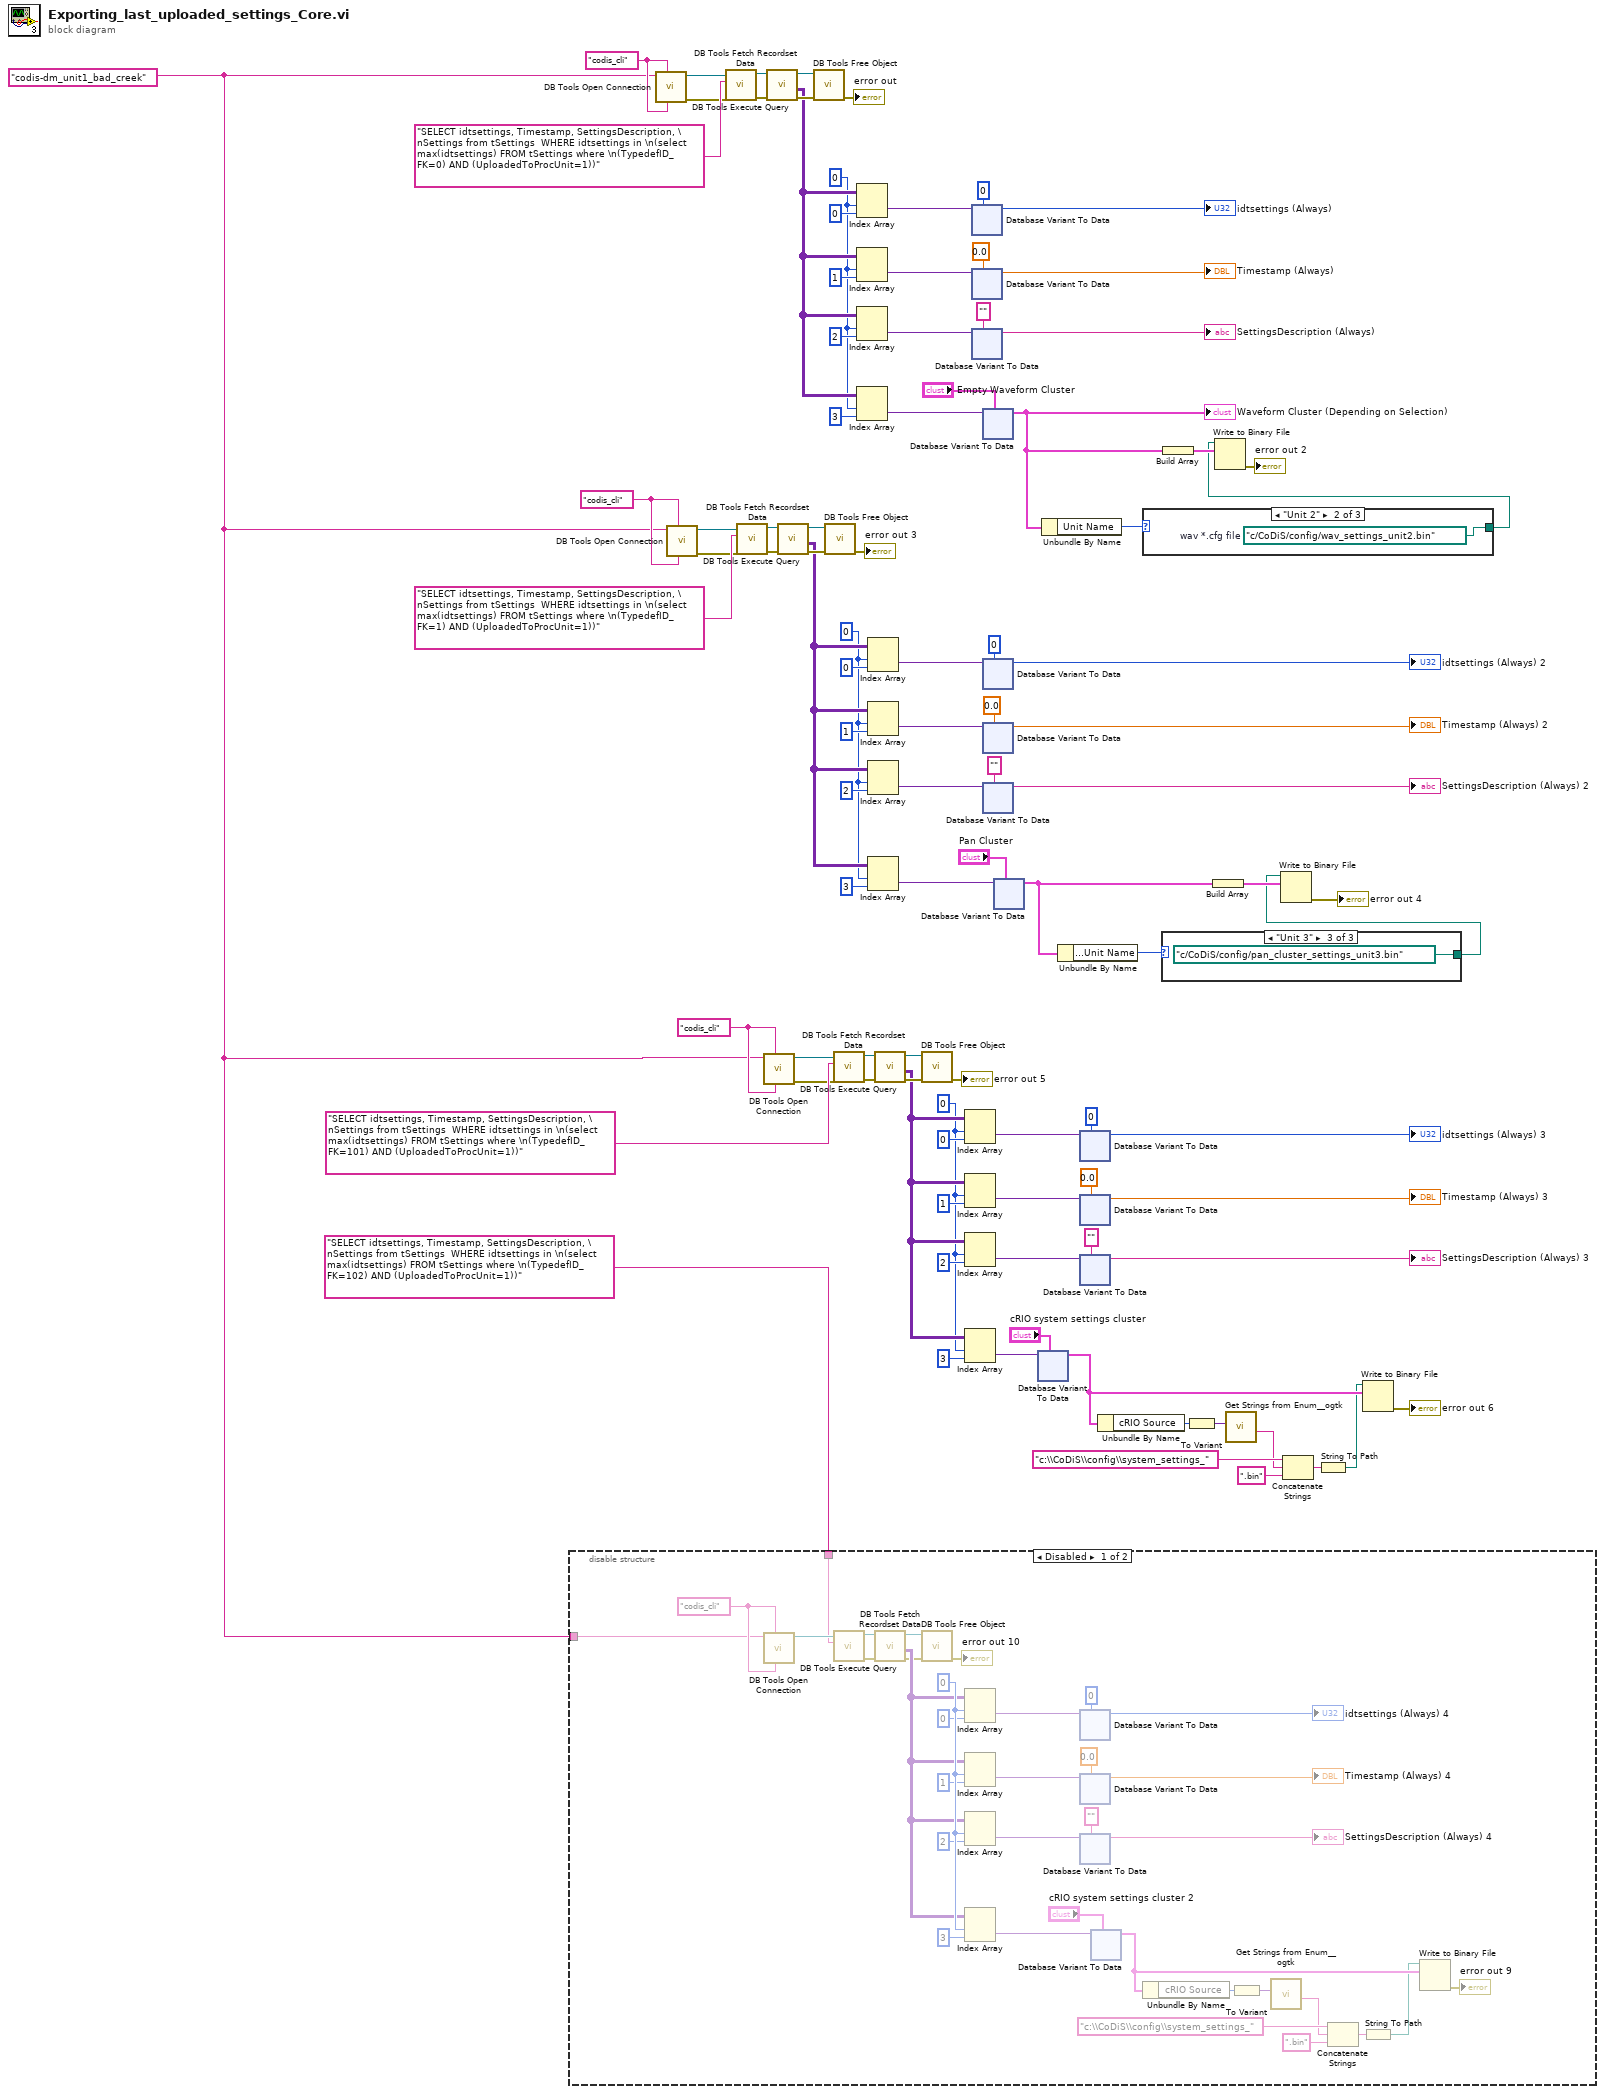
[diagram p0: block diagram]
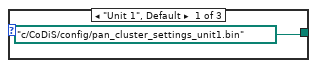
[diagram p3: hidden frame]
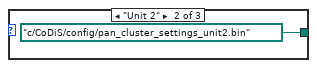
[diagram p4: hidden frame]
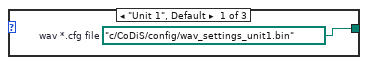
[diagram p5: hidden frame]
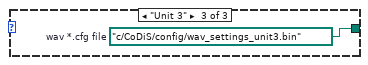
[diagram p6: hidden frame]
diagram:
  w13 = "codis-dm_unit1_bad_creek" ("userID")
  w26 = "codis_cli" ("userID")
  w33 = 0 ("disabled index (row)")
  w52 = "codis_cli" ("userID")
  w59 = 0 ("disabled index (row)")
  w78 = "codis_cli" ("userID")
  w85 = 0 ("disabled index (row)")
  n1 = disable-structure shown="Disabled" {
    disable-tunnel: w13 -> [w109 _]
    disable-tunnel: "SELECT idtsettings, Timestamp, SettingsDescription, \nSettings from tSettings  WHERE idtsettings in \n(select max(idtsettings) FROM tSettings where \n(TypedefID_FK=102) AND (UploadedToProcUnit=1))" -> [w108 _]
    frame Disabled {
      w130 = "codis_cli" ("userID")
      w123 = 0 ("disabled index (row)")
      n2 = call-poly <vilib>:"DB Tools Open Connection.vi"("password"=w130, "userID"=w130, "connection information"=w109) -> ("connection reference"=w131:T13)  [unwired: 5 in, 1 out]
      n3 = call-poly <vilib>:"DB Tools Execute Query.vi"("SQL query"=w108, "connection reference"=w131) -> ("error out"=w113:errorcluster, "recordset reference"=w114:T14)  [unwired: 6 in]
      n4 = call-poly <vilib>:"DB Tools Fetch Recordset Data.vi"("error in (no error)"=w113, "recordset reference"=w114) -> ("error out"=w116:errorcluster, "recordset data"=w122:variant[][], "recordset reference out"=w115:T14)  [unwired: 3 in]
      n5 = call-poly <vilib>:"DB Tools Free Object.vi"("error in (no error)"=w116, "recordset reference"=w115) -> ("error out"=→"error out 10":errorcluster)  [unwired: 8 in, 1 out]
      n6 = Index Array(array=w122, index (row)=w123, index (col)=0 ("index (row)")) -> (element=w124:variant)
      n7 = Index Array(array=w122, index (row)=w123, index (col)=1 ("index (row)")) -> (element=w126:variant)
      n8 = Index Array(array=w122, index (row)=w123, index (col)=2 ("index (row)")) -> (element=w125:variant)
      n9 = Index Array(array=w122, index (row)=w123, index (col)=3 ("index (row)")) -> (element=w118:variant)
      n10 = xnode "Database Variant To Data"("database variant"=w124, "type"=u32 0) -> ("data"=→"idtsettings (Always) 4":u32)  [unwired: 1 in, 1 out]
      n11 = xnode "Database Variant To Data"("database variant"=w126, "type"=0.0) -> ("data"=→"Timestamp (Always) 4":dbl)  [unwired: 1 in, 1 out]
      n12 = xnode "Database Variant To Data"("database variant"=w125, "type"="") -> ("data"=→"SettingsDescription (Always) 4":string)  [unwired: 1 in, 1 out]
      n13 = xnode "Database Variant To Data"("database variant"=w118, "type"="cRIO system settings cluster 2") -> ("data"=w107:T1)  [unwired: 1 in, 1 out]
      n14 = Unbundle By Name(w107) -> ("cRIO Source"=w106:T3)
      n15 = To Variant(anything=w106) -> (Variant=w105:variant)
      n16 = call <userlib>:"Get Strings from Enum__ogtk.vi"("Enum"=w105) -> ("String Value"=w103:string)  [unwired: 7 in, 3 out]
      n17 = Concatenate Strings("c:\\CoDiS\\config\\system_settings_", w103, ".bin" ("string")) -> (w101:string)
      n18 = String To Path(string=w101) -> (path=w100:path)
      n19 = Write to Binary File(file (use dialog)=w100, data=w107) -> (error out=→"error out 9":errorcluster)  [unwired: 4 in, 2 out]
    }
    frame Enabled {
    }
  }
  n20 = call-poly <vilib>:"DB Tools Open Connection.vi"("password"=w78, "userID"=w78, "connection information"=w13) -> ("error out"=w3:errorcluster, "connection reference"=w77:T13)  [unwired: 5 in]
  n21 = call-poly <vilib>:"DB Tools Open Connection.vi"("password"=w52, "userID"=w52, "connection information"=w13) -> ("error out"=w2:errorcluster, "connection reference"=w51:T13)  [unwired: 5 in]
  n22 = call-poly <vilib>:"DB Tools Execute Query.vi"("error in (no error)"=w3, "SQL query"="SELECT idtsettings, Timestamp, SettingsDescription, \nSettings from tSettings  WHERE idtsettings in \n(select max(idtsettings) FROM tSettings where \n(TypedefID_FK=0) AND (UploadedToProcUnit=1))", "connection reference"=w77) -> ("error out"=w95:errorcluster, "recordset reference"=w94:T14)  [unwired: 5 in]
  n23 = call-poly <vilib>:"DB Tools Execute Query.vi"("error in (no error)"=w2, "SQL query"="SELECT idtsettings, Timestamp, SettingsDescription, \nSettings from tSettings  WHERE idtsettings in \n(select max(idtsettings) FROM tSettings where \n(TypedefID_FK=1) AND (UploadedToProcUnit=1))", "connection reference"=w51) -> ("error out"=w69:errorcluster, "recordset reference"=w68:T14)  [unwired: 5 in]
  n24 = call-poly <vilib>:"DB Tools Open Connection.vi"("password"=w26, "userID"=w26, "connection information"=w13) -> ("error out"=w1:errorcluster, "connection reference"=w25:T13)  [unwired: 5 in]
  n25 = call-poly <vilib>:"DB Tools Fetch Recordset Data.vi"("error in (no error)"=w95, "recordset reference"=w94) -> ("error out"=w92:errorcluster, "recordset data"=w86:variant[][], "recordset reference out"=w93:T14)  [unwired: 3 in]
  n26 = call-poly <vilib>:"DB Tools Fetch Recordset Data.vi"("error in (no error)"=w69, "recordset reference"=w68) -> ("error out"=w66:errorcluster, "recordset data"=w60:variant[][], "recordset reference out"=w67:T14)  [unwired: 3 in]
  n27 = call-poly <vilib>:"DB Tools Free Object.vi"("error in (no error)"=w92, "recordset reference"=w93) -> ("error out"=→"error out":errorcluster)  [unwired: 8 in, 1 out]
  n28 = call-poly <vilib>:"DB Tools Free Object.vi"("error in (no error)"=w66, "recordset reference"=w67) -> ("error out"=→"error out 3":errorcluster)  [unwired: 8 in, 1 out]
  n29 = call-poly <vilib>:"DB Tools Execute Query.vi"("error in (no error)"=w1, "SQL query"="SELECT idtsettings, Timestamp, SettingsDescription, \nSettings from tSettings  WHERE idtsettings in \n(select max(idtsettings) FROM tSettings where \n(TypedefID_FK=101) AND (UploadedToProcUnit=1))", "connection reference"=w25) -> ("error out"=w43:errorcluster, "recordset reference"=w42:T14)  [unwired: 5 in]
  n30 = Index Array(array=w86, index (row)=w85, index (col)=0 ("index (row)")) -> (element=w84:variant)
  n31 = Index Array(array=w86, index (row)=w85, index (col)=1 ("index (row)")) -> (element=w82:variant)
  n32 = Index Array(array=w86, index (row)=w85, index (col)=2 ("index (row)")) -> (element=w83:variant)
  n33 = Index Array(array=w86, index (row)=w85, index (col)=3 ("index (row)")) -> (element=w90:variant)
  n34 = Index Array(array=w60, index (row)=w59, index (col)=0 ("index (row)")) -> (element=w58:variant)
  n35 = Index Array(array=w60, index (row)=w59, index (col)=1 ("index (row)")) -> (element=w56:variant)
  n36 = Index Array(array=w60, index (row)=w59, index (col)=2 ("index (row)")) -> (element=w57:variant)
  n37 = Index Array(array=w60, index (row)=w59, index (col)=3 ("index (row)")) -> (element=w64:variant)
  n38 = call-poly <vilib>:"DB Tools Fetch Recordset Data.vi"("error in (no error)"=w43, "recordset reference"=w42) -> ("error out"=w40:errorcluster, "recordset data"=w34:variant[][], "recordset reference out"=w41:T14)  [unwired: 3 in]
  n39 = call-poly <vilib>:"DB Tools Free Object.vi"("error in (no error)"=w40, "recordset reference"=w41) -> ("error out"=→"error out 5":errorcluster)  [unwired: 8 in, 1 out]
  n40 = Index Array(array=w34, index (row)=w33, index (col)=0 ("index (row)")) -> (element=w32:variant)
  n41 = Index Array(array=w34, index (row)=w33, index (col)=1 ("index (row)")) -> (element=w30:variant)
  n42 = Index Array(array=w34, index (row)=w33, index (col)=2 ("index (row)")) -> (element=w31:variant)
  n43 = Index Array(array=w34, index (row)=w33, index (col)=3 ("index (row)")) -> (element=w38:variant)
  n44 = xnode "Database Variant To Data"("database variant"=w84, "type"=u32 0) -> ("data"=→"idtsettings (Always)":u32)  [unwired: 1 in, 1 out]
  n45 = xnode "Database Variant To Data"("database variant"=w82, "type"=0.0) -> ("data"=→"Timestamp (Always)":dbl)  [unwired: 1 in, 1 out]
  n46 = xnode "Database Variant To Data"("database variant"=w83, "type"="") -> ("data"=→"SettingsDescription (Always)":string)  [unwired: 1 in, 1 out]
  n47 = xnode "Database Variant To Data"("database variant"=w90, "type"="Empty Waveform Cluster") -> ("data"=w17:T7)  [unwired: 1 in, 1 out]
  "Waveform Cluster (Depending on Selection)" <- w17
  n48 = xnode "Database Variant To Data"("database variant"=w58, "type"=u32 0) -> ("data"=→"idtsettings (Always) 2":u32)  [unwired: 1 in, 1 out]
  n49 = xnode "Database Variant To Data"("database variant"=w56, "type"=0.0) -> ("data"=→"Timestamp (Always) 2":dbl)  [unwired: 1 in, 1 out]
  n50 = xnode "Database Variant To Data"("database variant"=w57, "type"="") -> ("data"=→"SettingsDescription (Always) 2":string)  [unwired: 1 in, 1 out]
  n51 = xnode "Database Variant To Data"("database variant"=w64, "type"="Pan Cluster") -> ("data"=w19:T4)  [unwired: 1 in, 1 out]
  n52 = xnode "Database Variant To Data"("database variant"=w38, "type"="cRIO system settings cluster") -> ("data"=w5:T1)  [unwired: 1 in, 1 out]
  n53 = Unbundle By Name(w17) -> ("Unit Name"=w16:T6)
  n54 = Unbundle By Name(w19) -> ("Condition Vector Cluster.Unit Name"=w15:T6)
  n55 = xnode "Database Variant To Data"("database variant"=w32, "type"=u32 0) -> ("data"=→"idtsettings (Always) 3":u32)  [unwired: 1 in, 1 out]
  n56 = xnode "Database Variant To Data"("database variant"=w30, "type"=0.0) -> ("data"=→"Timestamp (Always) 3":dbl)  [unwired: 1 in, 1 out]
  n57 = xnode "Database Variant To Data"("database variant"=w31, "type"="") -> ("data"=→"SettingsDescription (Always) 3":string)  [unwired: 1 in, 1 out]
  n58 = Unbundle By Name(w5) -> ("cRIO Source"=w11:T3)
  n59 = case shown="\"Unit 2\"" w16 {
    tunnel: [w266 w267 w268] -> w18
    frame "Unit 1", Default {
      w266 = path "c:/CoDiS/config/wav_settings_unit1.bin"  # wav *.cfg file
    }
    frame "Unit 2" {
      w267 = path "c:/CoDiS/config/wav_settings_unit2.bin"  # wav *.cfg file
    }
    frame "Unit 3" {
      w268 = path "c:/CoDiS/config/wav_settings_unit3.bin"  # wav *.cfg file
    }
  }
  n60 = case shown="\"Unit 3\"" w15 {
    tunnel: [path "c:/CoDiS/config/pan_cluster_settings_unit1.bin" ("file.tnd") path "c:/CoDiS/config/pan_cluster_settings_unit2.bin" ("file.tnd") path "c:/CoDiS/config/pan_cluster_settings_unit3.bin" ("file.tnd")] -> w14
    frame "Unit 1", Default {
    }
    frame "Unit 2" {
    }
    frame "Unit 3" {
    }
  }
  n61 = Build Array(w17) -> (w75:T7[])
  n62 = To Variant(anything=w11) -> (Variant=w10:variant)
  n63 = Build Array(w19) -> (w49:T4[])
  n64 = Write to Binary File(file (use dialog)=w18, data=w75) -> (error out=→"error out 2":errorcluster)  [unwired: 4 in, 2 out]
  n65 = call <userlib>:"Get Strings from Enum__ogtk.vi"("Enum"=w10) -> ("String Value"=w8:string)  [unwired: 7 in, 3 out]
  n66 = Write to Binary File(file (use dialog)=w14, data=w49) -> (error out=→"error out 4":errorcluster)  [unwired: 4 in, 2 out]
  n67 = Concatenate Strings("c:\\CoDiS\\config\\system_settings_", w8, ".bin" ("string")) -> (w6:string)
  n68 = String To Path(string=w6) -> (path=w4:path)
  n69 = Write to Binary File(file (use dialog)=w4, data=w5) -> (error out=→"error out 6":errorcluster)  [unwired: 4 in, 2 out]
